vi "RT_PID_Velocity.vi"() -> ()   [LabVIEW 2014]
uses:
  <vilib>/FPGAPlugInAG/cRIO-9068/niLvFpga_Open_cRIO-9068.vi
  <vilib>/rvi/interface/common/dynamic/niFpgaDynamicAddResources.vi
  <vilib>/Utility/error.llb/Error Cluster From Error Code.vi
  <vilib>/rvi/errors/niLvFpgaAdjustHostInterfaceError.vi
  <vilib>/addons/control/pid/pid.llb/PID (DBL).vi
  <vilib>/FPGAPlugInAG/Dynamic/niLvFpga_Close_Dynamic.vi
  <vilib>/rvi/interface/nirviOpenFPGA/nirviOpenFPGA.xnode
  FPGA Bitfiles/Motortest_FPGATarget_test6auto_Jx62XASY7Q8.lvbitx
  <vilib>/rvi/interface/nirviReadWriteControl/nirviReadWriteControl.xnode
  <vilib>/rvi/interface/nirviCloseFPGA/nirviCloseFPGA.xnode
  NiFpgaLv.dll
  <vilib>/rvi/interface/Simulation/niFpgaSimulationCallBeginRW.vi
  <vilib>/addons/control/pid/NI_PID_pid.lvlib
panel:
  out "Duty Cycle":dbl(slide) scale=0.0..1.0
  out "Error":dbl(slide) scale=0.0..50.0
  out "Velocity":sgl[](graph)
  out "Duty Cycle":dbl[](graph)
  out "Duty Cycle":dbl format="%.2f"
  in  "output range":cluster{"output high":dbl, "output low":dbl}={"output high"=100.0, "output low"=-100.0} {"output low" format="%.2f"; "output high" format="%.2f"}
  in  "PID gains":T1={"proportional gain (Kc)"=0.15, "integral time (Ti, min)"=0.0002, "derivative time (Td, min)"=0.0} {"derivative time (Td, min)" format="%.4f"; "integral time (Ti, min)" format="%.4f"; "proportional gain (Kc)" format="%.4f"}
  in  "Desired Velocity":dbl=30.0 format="%.2f"
  out "Velocity [RPS]":sgl
  out "Position [Round]":sgl
  in  "stop":bool
  # "Error"
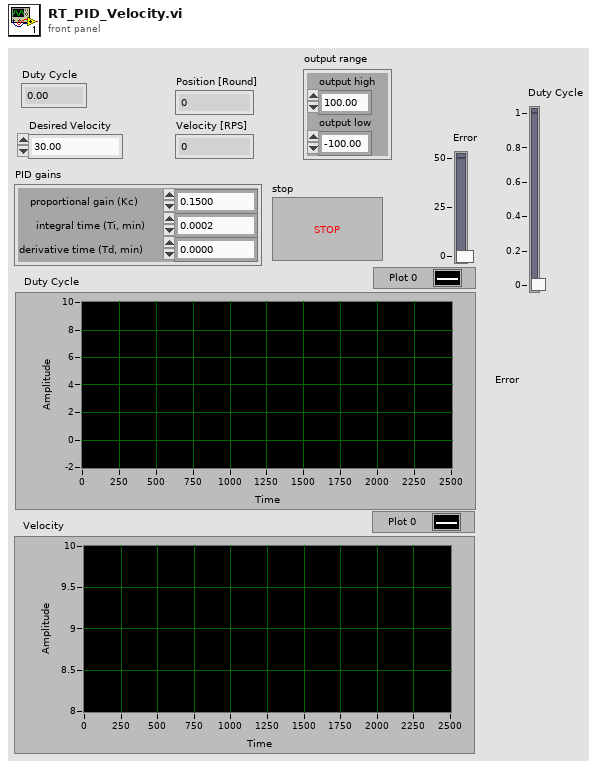
[diagram p1: front panel]
types:
  T1 = cluster{"proportional gain (Kc)":dbl, "integral time (Ti, min)":dbl, "derivative time (Td, min)":dbl}
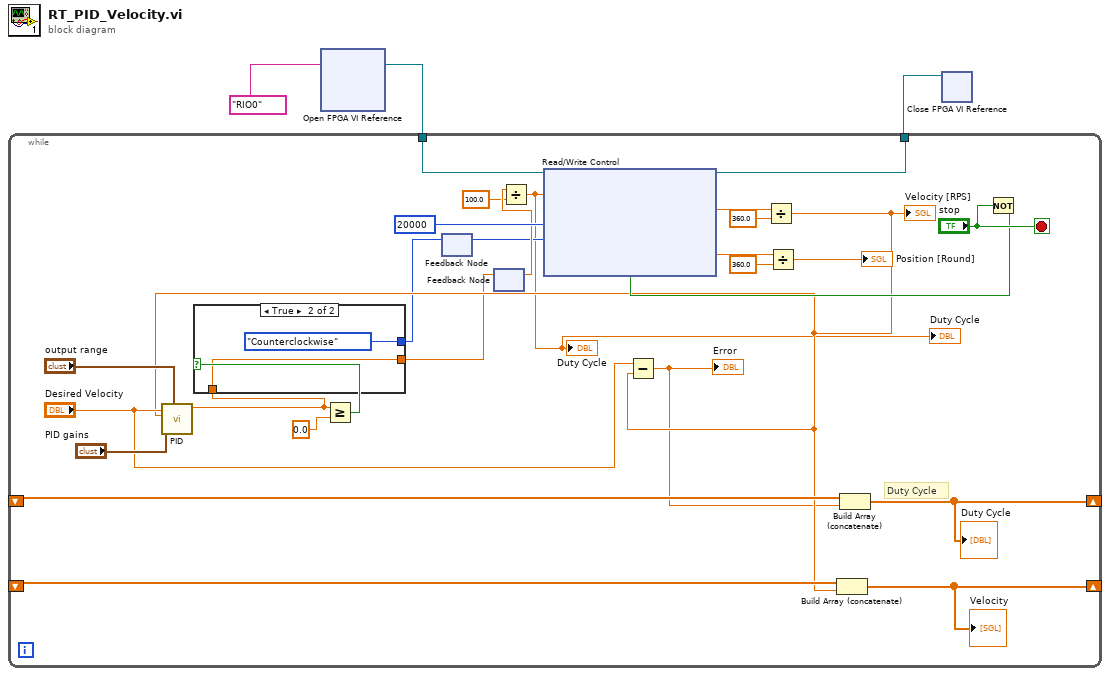
[diagram p0: block diagram]
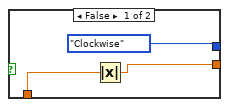
[diagram p2: hidden frame]
diagram:
  n1 = xnode "Open FPGA VI Reference"("resource name"=tag "RIO0") -> ("FPGA VI Reference Out"=w1:refnum<k20>)  [unwired: 1 in, 1 out]
  n2 = while {
    tunnel: w1 -> [w31]
    tunnel: [w30] -> w3
    shift-right: [w20] -> _
    shift-left: _ -> [w21]
    shift-right: [w4] -> _
    shift-left: _ -> [w19]
    stop <- "stop" stop-if-true
    # "Duty Cycle"
    n3 = feedback #1() -> (w7:enum8{"Clockwise", "Counterclockwise"})  [unwired: 1 in]
    n4 = feedback #2() -> (w15:dbl)  [unwired: 1 in]
    n5 = Divide(x=w15, y=100.0) -> (x/y=w5:dbl)
    "Duty Cycle" <- w5
    "Duty Cycle" <- w5
    n6 = Not(x="stop") -> (.not. x?=w28:bool)
    n7 = xnode "Read/Write Control"("FPGA VI Reference In"=w31, "duty cycle (periods)"=w5, "Velocity Interval (uSec)"=u32 20000, "Mod1/Drive Direction"=w7, "Mod1/Motor"=w28) -> ("FPGA VI Reference Out"=w30:refnum<k20>, "Velocity (Degrees/Second)"=w17:sgl, "Position (Degrees)"=w24:sgl)  [unwired: 1 in, 1 out]
    n8 = Divide(x=w17, y=sgl 360.0) -> (x/y=w13:sgl)
    "Velocity [RPS]" <- w13
    n9 = call-poly <vilib>:"PID.vi"("output range"="output range", "PID gains"="PID gains", "process variable"=w13, "setpoint"="Desired Velocity") -> ("output"=w10:dbl)  [unwired: 6 in, 1 out]
    n10 = Greater Or Equal?(x=w10, y=0.0) -> (x >= y?=w11:bool)
    n11 = case shown="True" w11 {
      tunnel: w10 -> [w32 w36]
      tunnel: [w33 w36] -> w9
      tunnel: [enum8{"Clockwise", "Counterclockwise"}."Clockwise" ("Mod1/Drive Direction") enum8{"Clockwise", "Counterclockwise"}."Counterclockwise" ("Mod1/Drive Direction")] -> w8
      frame False {
        n12 = Absolute Value(x=w32) -> (abs(x)=w33:dbl)
      }
      frame True {
      }
    }
    n13 = feedback-in #1(w8) -> ()
    n14 = feedback-in #2(w9) -> ()
    n15 = Subtract(x="Desired Velocity", y=w13) -> (x-y=w6:dbl)
    "Error" <- w6
    n16 = Divide(x=w24, y=sgl 360.0) -> (x/y=→"Position [Round]":sgl)
    n17 = Build Array (concatenate)(w19, w13) -> (w4:sgl[])
    "Velocity" <- w4
    n18 = Build Array (concatenate)(w21, w6) -> (w20:dbl[])
    "Duty Cycle" <- w20
  }
  n19 = xnode "Close FPGA VI Reference"("FPGA VI Reference In"=w3) -> ()  [unwired: 1 in, 1 out]
